vi "PWM_Motor_Array.vi"(10 "Geschwindigkeit\nmultiplikator":dbl(knob)=0.1402796355699434 scale=0.0..1.0, 11 "PWM Sensor":dbl) -> (3 "PWM Motor":dbl)   [LabVIEW 2016]
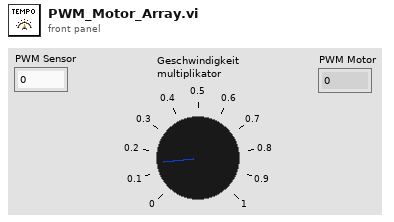
[diagram p1: front panel]
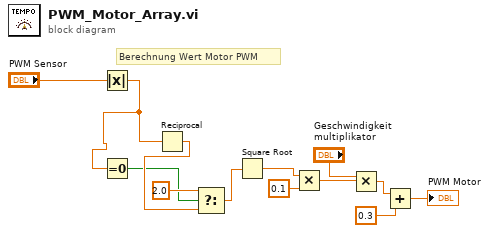
[diagram p0: block diagram]
diagram:
  # "Berechnung Wert Motor PWM"
  n1 = Absolute Value(x="PWM Sensor") -> (abs(x)=w1:dbl)
  n2 = Equal To 0?(x=w1) -> (x = 0?=w2:bool)
  n3 = Reciprocal(x=w1) -> (1/x=w6:dbl)
  n4 = Select(t=2.0, s=w2, f=w6) -> (s? t:f=w10:dbl)
  n5 = Square Root(x=w10) -> (sqrt(x)=w11:dbl)
  n6 = Multiply(x=w11, y=0.1) -> (x*y=w7:dbl)
  n7 = Multiply(x="Geschwindigkeit\nmultiplikator", y=w7) -> (x*y=w9:dbl)
  n8 = Add(x=w9, y=0.3) -> (x+y=→"PWM Motor":dbl)
